vi "Project_and_Mlink Template Creation.vi"(0 "Project Path":path=path "D:/Reference Architecture/Test.lvproj", 5 "Description":string, 11 "error in (no error)":errorcluster) -> (15 "error out":errorcluster)   [LabVIEW 2021, in "Migrator.lvlib"]
uses:
  Migrator.lvlib
  Measurement Plugin Generator/_Editor/MeasurementService Editor.lvlib
  Path Functions/Path Functions.lvlib
  Migrator Reusables/Migrator Reusables.lvlib
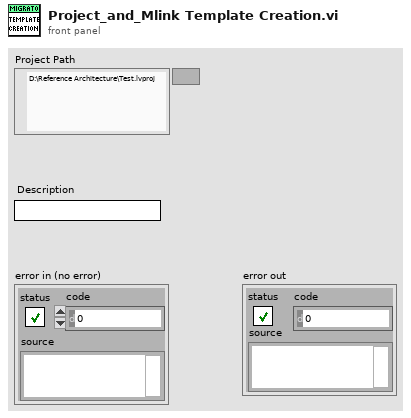
[diagram p1: front panel]
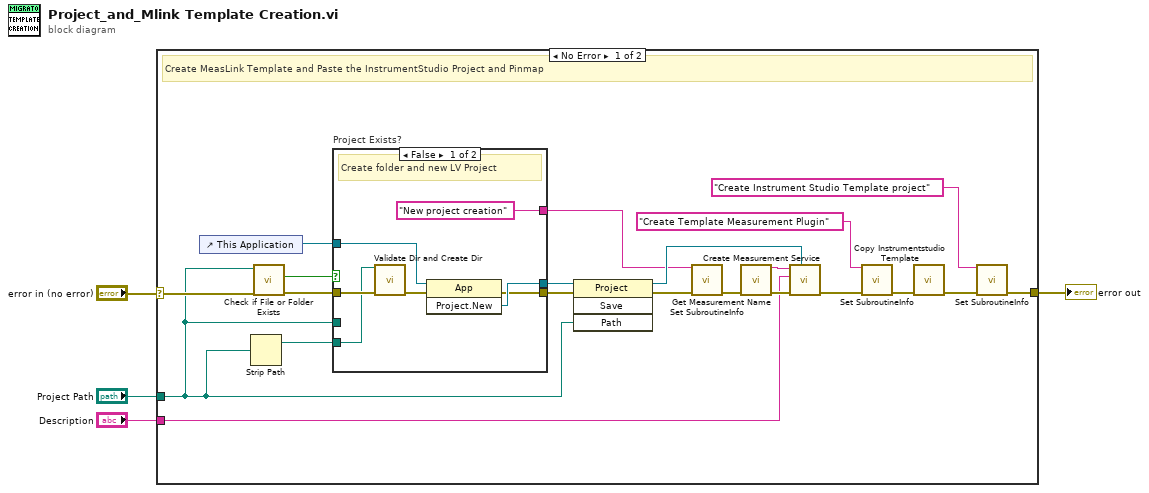
[diagram p0: block diagram]
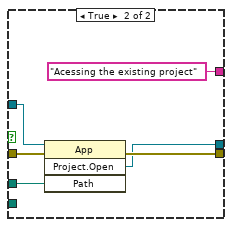
[diagram p2: hidden frame]
diagram:
  n1 = case shown="No Error" "error in (no error)" {
    selector: "error in (no error)" -> [w24 w39]
    tunnel: "Project Path" -> [w21 _]
    tunnel: [w6 w39] -> w2
    tunnel: "Description" -> [w16 _]
    frame No Error {
      # "Create MeasLink Template and Paste the InstrumentStudio Project and Pinmap"
      n2 = control-ref of="This Application"() -> (w20:refnum<vi>)
      n3 = Strip Path(path=w21) -> (stripped path=w25:path)  [unwired: 1 out]
      n4 = call <vilib>:"Check if File or Folder Exists.vi"("error in (no error)"=w24, "path"=w21) -> ("error out"=w23:errorcluster, "file or folder exists?"=w22:bool)  [unwired: 7 in, 1 out]
      n5 = case "Project Exists?" shown="False" w22 {
        tunnel: [w32 w35] -> w15
        tunnel: [w31 w36] -> w14
        tunnel: w25 -> [w28 _]
        tunnel: w23 -> [w29 w38]
        tunnel: w21 -> [_ w37]
        tunnel: w20 -> [w30 w34]
        tunnel: ["New project creation" ("Subroutine In") "Acessing the existing project" ("Subroutine In")] -> w11
        frame False {
          # "Create folder and new LV Project"
          n6 = call "Validate Dir and Create Dir.vi"("Directory"=w28, "error in (no error)"=w29) -> ("error out"=w27:errorcluster)  [unwired: 12 in, 1 out]
          n7 = invoke class="App" method="Project.New"(reference=w30, error in=w27) -> (error out=w31:errorcluster, "Project:New"=w32:refnum<vi>)  [unwired: 1 in, 1 out]
        }
        frame True {
          n8 = invoke class="App" method="Project.Open"(reference=w34, error in=w38, "Path"=w37) -> (error out=w36:errorcluster, "Project:Open"=w35:refnum<vi>)  [unwired: 1 in, 2 out]
        }
      }
      n9 = invoke class="Project" method="Save"(reference=w15, error in=w14, "Path"=w21) -> (reference out=w19:refnum<vi>, error out=w13:errorcluster)  [unwired: 1 in, 2 out]
      n10 = call "Set SubroutineInfo.vi"("Subroutine In"=w11, "error in (no error)"=w13) -> ("error out"=w12:errorcluster)  [unwired: 13 in]
      n11 = call "Get Measurement Name.vi"("error in (no error)"=w12) -> ("Name Out"=w17:string, "error out"=w18:errorcluster)  [unwired: 13 in]
      n12 = call "Create Measurement Service.vi"("project ref"=w19, "error in (no error)"=w18, "measurement plug-in description"=w16, "measurement plug-in name"=w17) -> ("error out"=w10:errorcluster)  [unwired: 7 in]
      n13 = call "Set SubroutineInfo.vi"("Subroutine In"="Create Template Measurement Plugin", "error in (no error)"=w10) -> ("error out"=w9:errorcluster)  [unwired: 13 in]
      n14 = call "Copy Instrumentstudio Template.vi"("error in (no error)"=w9) -> ("error out"=w7:errorcluster)  [unwired: 10 in]
      n15 = call "Set SubroutineInfo.vi"("Subroutine In"="Create Instrument Studio Template project", "error in (no error)"=w7) -> ("error out"=w6:errorcluster)  [unwired: 13 in]
    }
    frame Error {
    }
  }
  "error out" <- w2
